vi "ConfigureHighRateAnalysis.vi"(8 "error in (no error)":errorcluster) -> (0 "error out":errorcluster, 2 "register startup trends":T1[](array[typedef]), 3 "analysis config":T3, 5 "all config found?":bool)   [LabVIEW 2017, in "McsaAnalysisHighRate.lvlib"]
uses:
  <vilib>/addons/InsightCM/Devices/Shared/Mcsa/McsaAnalysisHighRate/McsaAnalysisHighRate.lvlib
  <vilib>/addons/InsightCM/Devices/Shared/Mcsa/McsaAnalysisHighRate/controls/Config.ctl
  <vilib>/addons/InsightCM/Devices/Shared/Mcsa/McsaAnalysisHighRate/controls/Group.ctl
  <vilib>/addons/InsightCM/Utilities/Analysis/MCSA/controls/McsaChannel.ctl
  <vilib>/addons/InsightCM/Utilities/Analysis/Shared/controls/Feature.ctl
  <vilib>/addons/InsightCM/Utilities/Analysis/Shared/controls/AmplitudeScale.ctl
  <vilib>/addons/InsightCM/MessageBus/Base/controls/KeyValuePair.ctl
  <vilib>/addons/InsightCM/Utilities/Analysis/MCSA/controls/McsaMotor.ctl
  <vilib>/addons/InsightCM/Devices/Shared/Common/DataEventCreator/controls/RegisterTrendPoints.ctl
  <vilib>/addons/InsightCM/Devices/Shared/Common/DataEventCreator/controls/Registry_Trend.ctl
  <vilib>/addons/InsightCM/Utilities/GlobalConfiguration/GlobalConfiguration.lvlib
  <vilib>/addons/InsightCM/Utilities/DeviceModelHelpers/DeviceModelHelpers.lvlib
  <vilib>/addons/InsightCM/Utilities/Analysis/Shared/AnalysisHelper.lvlib
  <vilib>/addons/InsightCM/Devices/Shared/Mcsa/McsaVirtualChannel/McsaVirtualChannel.lvlib
  <vilib>/addons/InsightCM/Utilities/Analysis/MCSA/McsaAnalysisFunctions.lvlib
  <vilib>/addons/InsightCM/Devices/Shared/Common/DataEventCreator/DataEventCreator.lvlib
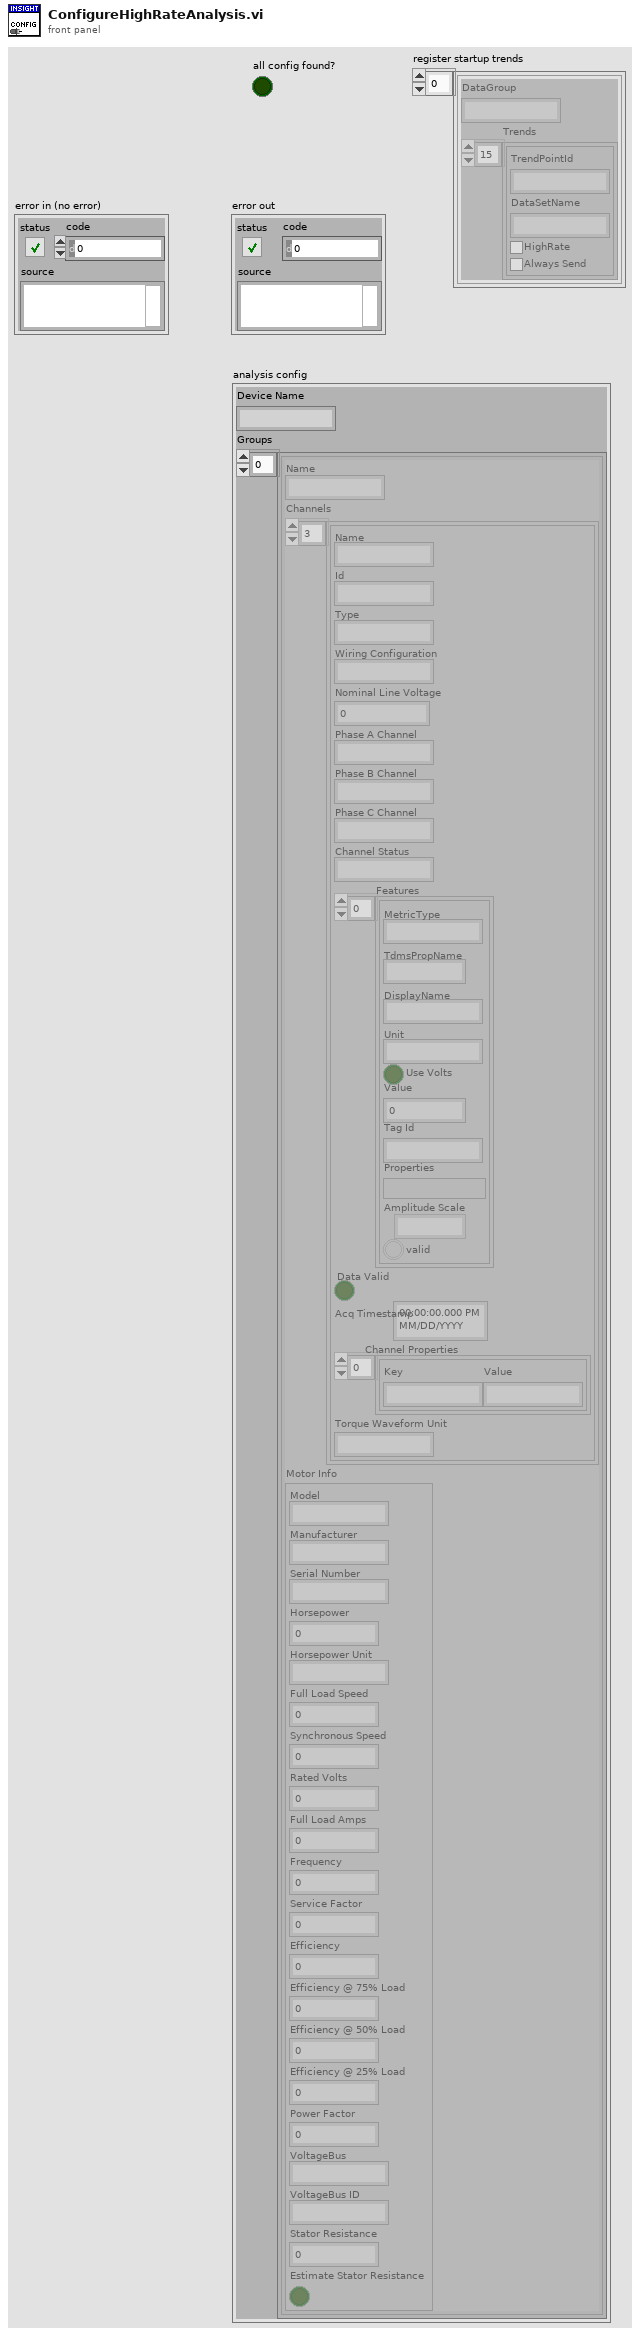
[diagram p1: front panel]
types:
  T1 = typedef "DataEventCreator.lvlib/RegisterTrendPoints.ctl" = cluster{"DataGroup":string, "Trends":T2[]}
  T2 = typedef "DataEventCreator.lvlib/Registry_Trend.ctl" = cluster{"TrendPointId":string, "DataSetName":string, "HighRate":bool, "Always Send":bool}
  T3 = typedef "McsaAnalysisHighRate.lvlib/Config.ctl" = cluster{"Device Name":string, "Groups":T4[]}
  T4 = typedef "McsaAnalysisHighRate.lvlib/Group.ctl" = cluster{"Name":string, "Channels":T5[], "Motor Info":T9}
  T5 = typedef "McsaAnalysisFunctions.lvlib/McsaChannel.ctl" = cluster{"Name":string, "Id":string, "Type":string, "Wiring Configuration":string, "Nominal Line Voltage":dbl, "Phase A Channel":string, "Phase B Channel":string, "Phase C Channel":string, "Channel Status":string, "Features":T6[], "Data Valid":bool, "Acq Timestamp":timestamp, "Channel Properties":T8[], "Torque Waveform Unit":string}
  T6 = typedef "AnalysisHelper.lvlib/Feature.ctl" = cluster{"MetricType":string, "TdmsPropName":string, "DisplayName":string, "Unit":string, "Use Volts":bool, "Value":dbl, "Tag Id":string, "Properties":variant, "Amplitude Scale":T7, "valid":bool}
  T7 = typedef "AnalysisHelper.lvlib/AmplitudeScale.ctl" = enum16{"rms", "peak", "pk-pk"}
  T8 = typedef "KeyValuePair.ctl" = cluster{"Key":string, "Value":string}
  T9 = typedef "McsaAnalysisFunctions.lvlib/McsaMotor.ctl" = cluster{"Model":string, "Manufacturer":string, "Serial Number":string, "Horsepower":dbl, "Horsepower Unit":string, "Full Load Speed":dbl, "Synchronous Speed":dbl, "Rated Volts":dbl, "Full Load Amps":dbl, "Frequency":dbl, "Service Factor":dbl, "Efficiency":dbl, "Efficiency @ 75% Load":dbl, "Efficiency @ 50% Load":dbl, "Efficiency @ 25% Load":dbl, "Power Factor":dbl, "VoltageBus":string, "VoltageBus ID":string, "Stator Resistance":dbl, "Estimate Stator Resistance":bool}
  T10 = typedef "R2_DeviceModel.ctl" = cluster{"Device":T11, "Channels":T18[], "Tags":T20[]}
  T11 = typedef "R2_Device.ctl" = cluster{"Id":string, "Name":string, "DeviceType":string, "HardwareName":string, "IpAddress":string, "HardwareInfo":T8[], "ApplicationType":string, "ApplicationVersion":string, "EquipmentIds":string[], "ConfigurationVersion":string, "State":T12, "Properties":T8[], "DataGroups":T13[], "BurstModeTrigger":T17}
  T12 = typedef "DeviceState.ctl" = cluster{"Disabled":bool}
  T13 = typedef "R2_DataGroup.ctl" = cluster{"Name":string, "OperatingStates":T14[], "Properties":T8[], "EquipmentIds":string[], "AssetNodeId":string}
  T14 = typedef "OperatingState.ctl" = cluster{"Name":string, "Properties":T8[], "Triggers":T15[]}
  T15 = typedef "Trigger.ctl" = cluster{"Type":string, "Expression":string, "Conditions":T16[]}
  T16 = typedef "Condition.ctl" = cluster{"Source":string, "Type":string, "Operator":string, "CompareTo":string, "DwellSeconds":dbl}
  T17 = typedef "BurstModeTrigger.ctl" = cluster{"Trigger":T15, "SampleRate":string, "AcquisitionLength":string}
  T18 = typedef "R2_Channel.ctl" = cluster{"Id":string, "DeviceId":string, "Name":string, "ChannelType":string, "HardwareKey":string, "HardwareChannel":string, "DataGroup":string, "Keywords":string[], "EquipmentIds":string[], "Properties":T8[], "Metrics":T19[], "AssetNodeId":string, "MeasType":string, "AssetName":string}
  T19 = typedef "Metric.ctl" = cluster{"Id":string, "Name":string, "Unit":string, "Properties":T8[], "MetricDefinitionInstanceId":string}
  T20 = typedef "Tag.ctl" = cluster{"Id":string, "Path":string, "Name":string, "Datatype":string, "Props":T8[], "Keywords":string[]}
  T21 = typedef "SectionKeyValues.ctl" = cluster{"Section":string, "KeyValues":T8[]}
  T22 = typedef "MetricDefinitionInstance.ctl" = cluster{"Id":string, "MetricType":string, "Name":string, "Properties":T8[], "HighRate":bool}
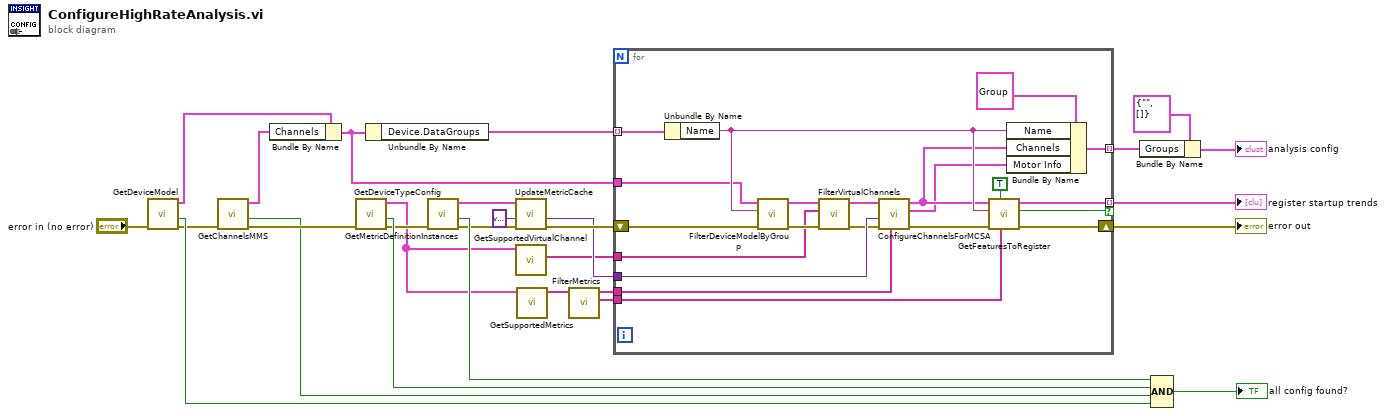
[diagram p0: block diagram]
diagram:
  n1 = call <vilib>:"GetDeviceModel.vi"("error in (no error)"="error in (no error)") -> ("error out"=w5:errorcluster, "found"=w23:bool, "device model"=w7:T10)  [unwired: 8 in]
  n2 = call <vilib>:"GetChannelsMMS.vi"("error in (no error)"=w5) -> ("error out"=w4:errorcluster, "found"=w2:bool, "MMS Channels"=w3:T18[])  [unwired: 6 in, 2 out]
  n3 = Bundle By Name(cluster=w7, "Channels"=w3) -> (w6:T10)
  n4 = call <vilib>:"GetDeviceTypeConfig.vi"("error in (no error)"=w4) -> ("error out"=w13:errorcluster, "found"=w21:bool, "key values"=w12:T21[])  [unwired: 8 in]
  n5 = Unbundle By Name(w6) -> ("Device.DataGroups"=w28:T13[])
  n6 = call <vilib>:"GetMetricDefinitionInstances.vi"("error in (no error)"=w13) -> ("error out"=w19:errorcluster, "found"=w22:bool, "metrics"=w17:T22[])  [unwired: 8 in]
  n7 = call <vilib>:"UpdateMetricCache.vi"("error in (no error)"=w19, "Metrics"=variant, "MetricDefinitionInstances"=w17) -> ("error out"=w18:errorcluster, "Metrics out"=w16:variant)  [unwired: 7 in]
  n8 = call <vilib>:"GetSupportedVirtualChannel.vi"("key values"=w12) -> ("not supported virtual channels"=w11:string[])  [unwired: 9 in, 1 out]
  n9 = call <vilib>:"GetSupportedMetrics.vi"("key values"=w12) -> ("supported metrics"=w10:string[])  [unwired: 10 in]
  n10 = call <vilib>:"FilterMetrics.vi"("supported metrics"=w10) -> ("startup metrics supported in data viewer"=w1:string[], "high rate calculation supported metrics"=w9:string[])  [unwired: 9 in]
  n11 = for {
    tunnel: w16 -> [w49]
    tunnel: w6 -> [w36]
    shift-right: [w46] -> w27
    shift-left: w18 -> [w47]
    tunnel: [w48] -> w14 mode=indexing
    tunnel: w28 -> [w34] mode=indexing
    tunnel: [w45] -> w26 mode=indexing if=w44
    tunnel: w9 -> [w31]
    tunnel: w11 -> [w37]
    tunnel: w1 -> [w30]
    n12 = Unbundle By Name(w34) -> ("Name"=w43:string)
    n13 = call <vilib>:"FilterDeviceModelByGroup.vi"("error in (no error)"=w47, "group"=w43, "device model"=w36) -> ("error out"=w38:errorcluster, "device model (channels filtered by group)"=w40:T10)  [unwired: 7 in]
    n14 = call <vilib>:"FilterVirtualChannels.vi"("error in (no error)"=w38, "not supported virtual channels"=w37, "device model"=w40) -> ("error out"=w39:errorcluster, "device model (unsupported virtual channels filtered out)"=w41:T10)  [unwired: 7 in]
    n15 = call <vilib>:"ConfigureChannelsForMCSA.vi"("Supported Metrics"=w31, "error in (no error)"=w39, "metric cache"=w49, "device"=w41) -> ("error out"=w42:errorcluster, "Motor Info Out"=w29:T9, "channels"=w32:T5[])  [unwired: 5 in]
    n16 = call <vilib>:"GetFeaturesToRegister.vi"("Supported Metrics"=w30, "high rate"=TRUE, "error in (no error)"=w42, "group"=w43, "channels"=w32) -> ("error out"=w46:errorcluster, "atleast one"=w44:bool, "register trend"=w45:T1)  [unwired: 4 in]
    n17 = Bundle By Name(cluster=T4 {"Name"="", "Channels"=[], "Motor Info"={"Model"="", "Manufacturer"="", "Serial Number"="", "Horsepower"=0.0, "Horsepower Unit"="", "Full Load Speed"=0.0, "Synchronous Speed"=0.0, "Rated Volts"=0.0, "Full Load Amps"=0.0, "Frequency"=0.0, "Service Factor"=0.0, "Efficiency"=0.0, "Efficiency @ 75% Load"=0.0, "Efficiency @ 50% Load"=0.0, "Efficiency @ 25% Load"=0.0, "Power Factor"=0.0, "VoltageBus"="", "VoltageBus ID"="", "Stator Resistance"=0.0, "Estimate Stator Resistance"=FALSE}} ("Group"), "Name"=w43, "Channels"=w32, "Motor Info"=w29) -> (w48:T4)
  }
  "error out" <- w27
  "register startup trends" <- w26
  n18 = Bundle By Name(cluster=T3 {"Device Name"="", "Groups"=[]} ("Analysis Configuration"), "Groups"=w14) -> (→"analysis config":T3)
  n19 = Compound Arithmetic op=AND(w22, w21, w2, w23) -> (→"all config found?":bool)
